vi "实时小时数据处理整合 (子VI).vi"(11 "枚举":enum16{"实时数据排序", "小时数据排序"}(ring)) -> (3 "已排序的数组":string[](array[string]))   [LabVIEW 2016]
uses:
  <userlib>/_OpenG.lib/array/array.llb/Remove Duplicates from 1D Array (String)__ogtk.vi
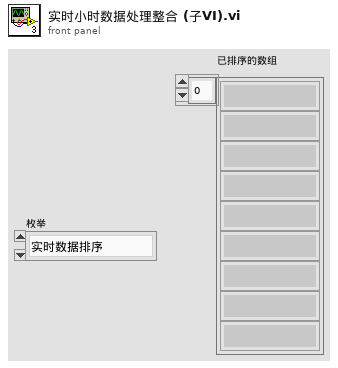
[diagram p1: front panel]
types:
  T1 = cluster{"PH":string[][], "CODCr":string[][], "氨氮":string[][], "CODMn":string[][], "总氮":string[][], "总磷":string[][], "电导率":string[][], "水温":string[][], "DO":string[][], "浊度":string[][], "叶绿素":string[][], "藻密度":string[][], "铜":string[][], "盐度":string[][], "水位":string[][], "流速":string[][], "瞬时流量":string[][], "累积流量":string[][]}
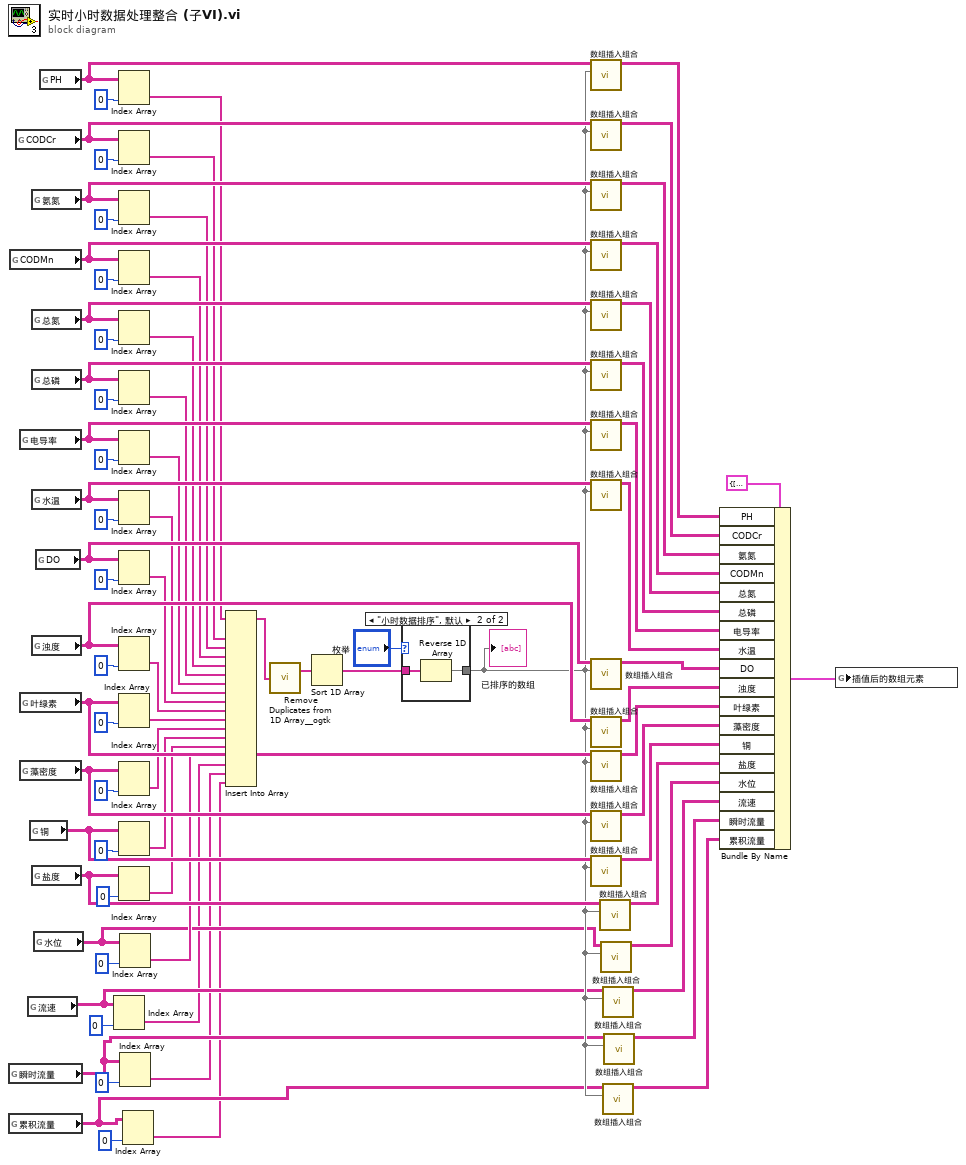
[diagram p0: block diagram]
diagram:
  n1 = global read "全局 所有参数.vi" "瞬时流量"() -> (w10:string[][])
  n2 = global read "全局 所有参数.vi" "累积流量"() -> (w9:string[][])
  n3 = global read "全局 所有参数.vi" "CODMn"() -> (w60:string[][])
  n4 = global read "全局 所有参数.vi" "CODCr"() -> (w58:string[][])
  n5 = global read "全局 所有参数.vi" "电导率"() -> (w63:string[][])
  n6 = global read "全局 所有参数.vi" "叶绿素"() -> (w67:string[][])
  n7 = global read "全局 所有参数.vi" "藻密度"() -> (w68:string[][])
  n8 = global read "全局 所有参数.vi" "流速"() -> (w14:string[][])
  n9 = global read "全局 所有参数.vi" "铜"() -> (w27:string[][])
  n10 = global read "全局 所有参数.vi" "氨氮"() -> (w59:string[][])
  n11 = global read "全局 所有参数.vi" "总氮"() -> (w61:string[][])
  n12 = global read "全局 所有参数.vi" "总磷"() -> (w62:string[][])
  n13 = global read "全局 所有参数.vi" "水温"() -> (w64:string[][])
  n14 = global read "全局 所有参数.vi" "浊度"() -> (w66:string[][])
  n15 = global read "全局 所有参数.vi" "盐度"() -> (w26:string[][])
  n16 = global read "全局 所有参数.vi" "水位"() -> (w16:string[][])
  n17 = global read "全局 所有参数.vi" "DO"() -> (w65:string[][])
  n18 = global read "全局 所有参数.vi" "PH"() -> (w56:string[][])
  n19 = Index Array(array=w14, index (col)=0 ("索引 (列)")) -> (element=w13:string[])  [unwired: 1 in]
  n20 = Index Array(array=w56, index (col)=0 ("索引 (行)")) -> (element=w43:string[])  [unwired: 1 in]
  n21 = Index Array(array=w58, index (col)=0 ("索引 (行)")) -> (element=w44:string[])  [unwired: 1 in]
  n22 = Index Array(array=w59, index (col)=0 ("索引 (行)")) -> (element=w45:string[])  [unwired: 1 in]
  n23 = Index Array(array=w60, index (col)=0 ("索引 (行)")) -> (element=w46:string[])  [unwired: 1 in]
  n24 = Index Array(array=w61, index (col)=0 ("索引 (行)")) -> (element=w47:string[])  [unwired: 1 in]
  n25 = Index Array(array=w62, index (col)=0 ("索引 (行)")) -> (element=w48:string[])  [unwired: 1 in]
  n26 = Index Array(array=w63, index (col)=0 ("索引 (行)")) -> (element=w49:string[])  [unwired: 1 in]
  n27 = Index Array(array=w64, index (col)=0 ("索引 (行)")) -> (element=w50:string[])  [unwired: 1 in]
  n28 = Index Array(array=w65, index (col)=0 ("索引 (行)")) -> (element=w51:string[])  [unwired: 1 in]
  n29 = Index Array(array=w66, index (col)=0 ("索引 (行)")) -> (element=w52:string[])  [unwired: 1 in]
  n30 = Index Array(array=w67, index (col)=0 ("索引 (行)")) -> (element=w53:string[])  [unwired: 1 in]
  n31 = Index Array(array=w68, index (col)=0 ("索引 (行)")) -> (element=w54:string[])  [unwired: 1 in]
  n32 = Index Array(array=w27, index (col)=0 ("索引 (行)")) -> (element=w25:string[])  [unwired: 1 in]
  n33 = Index Array(array=w26, index (col)=0 ("索引 (行)")) -> (element=w24:string[])  [unwired: 1 in]
  n34 = Index Array(array=w16, index (col)=0 ("索引 (列)")) -> (element=w17:string[])  [unwired: 1 in]
  n35 = Index Array(array=w10, index (col)=0 ("索引 (列)")) -> (element=w7:string[])  [unwired: 1 in]
  n36 = Index Array(array=w9, index (col)=0 ("索引 (列)")) -> (element=w8:string[])  [unwired: 1 in]
  n37 = Insert Into Array(array=w43, new element #1=w44, new element #2=w45, new element #3=w46, new element #4=w47, new element #5=w48, new element #6=w49, new element #7=w50, new element #8=w51, new element #9=w52, new element #10=w53, new element #11=w54, new element #12=w25, new element #13=w24, new element #14=w17, new element #15=w13, new element #16=w7, new element #17=w8) -> (w55:string[])  [unwired: 1 in]
  n38 = call-poly <userlib>:"Remove Duplicates from 1D Array__ogtk.vi"("Input Array"=w55) -> ("Output Array"=w42:string[])  [unwired: 1 out]
  n39 = Sort 1D Array(array=w42) -> (sorted array=w28:string[])
  n40 = case shown="\"小时数据排序\", 默认" "枚举" {
    tunnel: w28 -> [w80 w82]
    tunnel: [w80 w81] -> w19
    frame "实时数据排序" {
    }
    frame "小时数据排序", Default {
      n41 = Reverse 1D Array(array=w82) -> (reversed array=w81:string[])
    }
  }
  "已排序的数组" <- w19
  n42 = call "数组插入组合.vi"("排序后的一维数组"=w19, "输入数组"=w56) -> ("输出结果"=w57:string[][])  [unwired: 9 in]
  n43 = call "数组插入组合.vi"("排序后的一维数组"=w19, "输入数组"=w58) -> ("输出结果"=w69:string[][])  [unwired: 9 in]
  n44 = call "数组插入组合.vi"("排序后的一维数组"=w19, "输入数组"=w59) -> ("输出结果"=w70:string[][])  [unwired: 9 in]
  n45 = call "数组插入组合.vi"("排序后的一维数组"=w19, "输入数组"=w60) -> ("输出结果"=w71:string[][])  [unwired: 9 in]
  n46 = call "数组插入组合.vi"("排序后的一维数组"=w19, "输入数组"=w61) -> ("输出结果"=w72:string[][])  [unwired: 9 in]
  n47 = call "数组插入组合.vi"("排序后的一维数组"=w19, "输入数组"=w62) -> ("输出结果"=w73:string[][])  [unwired: 9 in]
  n48 = call "数组插入组合.vi"("排序后的一维数组"=w19, "输入数组"=w63) -> ("输出结果"=w74:string[][])  [unwired: 9 in]
  n49 = call "数组插入组合.vi"("排序后的一维数组"=w19, "输入数组"=w64) -> ("输出结果"=w75:string[][])  [unwired: 9 in]
  n50 = call "数组插入组合.vi"("排序后的一维数组"=w19, "输入数组"=w65) -> ("输出结果"=w76:string[][])  [unwired: 9 in]
  n51 = call "数组插入组合.vi"("排序后的一维数组"=w19, "输入数组"=w66) -> ("输出结果"=w77:string[][])  [unwired: 9 in]
  n52 = call "数组插入组合.vi"("排序后的一维数组"=w19, "输入数组"=w67) -> ("输出结果"=w78:string[][])  [unwired: 9 in]
  n53 = call "数组插入组合.vi"("排序后的一维数组"=w19, "输入数组"=w68) -> ("输出结果"=w79:string[][])  [unwired: 9 in]
  n54 = call "数组插入组合.vi"("排序后的一维数组"=w19, "输入数组"=w27) -> ("输出结果"=w23:string[][])  [unwired: 9 in]
  n55 = call "数组插入组合.vi"("排序后的一维数组"=w19, "输入数组"=w26) -> ("输出结果"=w22:string[][])  [unwired: 9 in]
  n56 = call "数组插入组合.vi"("排序后的一维数组"=w19, "输入数组"=w16) -> ("输出结果"=w6:string[][])  [unwired: 9 in]
  n57 = call "数组插入组合.vi"("排序后的一维数组"=w19, "输入数组"=w14) -> ("输出结果"=w5:string[][])  [unwired: 9 in]
  n58 = call "数组插入组合.vi"("排序后的一维数组"=w19, "输入数组"=w9) -> ("输出结果"=w3:string[][])  [unwired: 9 in]
  n59 = call "数组插入组合.vi"("排序后的一维数组"=w19, "输入数组"=w10) -> ("输出结果"=w4:string[][])  [unwired: 9 in]
  n60 = Bundle By Name(cluster=T1 {"PH"=[], "CODCr"=[], "氨氮"=[], "CODMn"=[], "总氮"=[], "总磷"=[], "电导率"=[], "水温"=[], "DO"=[], "浊度"=[], "叶绿素"=[], "藻密度"=[], "铜"=[], "盐度"=[], "水位"=[], "流速"=[], "瞬时流量"=[], "累积流量"=[]} ("插值后的数组元素"), "PH"=w57, "CODCr"=w69, "氨氮"=w70, "CODMn"=w71, "总氮"=w72, "总磷"=w73, "电导率"=w74, "水温"=w75, "DO"=w76, "浊度"=w77, "叶绿素"=w78, "藻密度"=w79, "铜"=w23, "盐度"=w22, "水位"=w6, "流速"=w5, "瞬时流量"=w4, "累积流量"=w3) -> (w1:T1)
  n61 = global write "插值后的新数组.vi" "插值后的数组元素"(w1) -> ()
